vi "Parse Next Socket CAN.vi"(8 "error in (no error)":errorcluster, 10 "CAN pcap in":u8[](array[numeric]), 11 "pcap Parse and Build in":refnum<class "pcap_Parse_Build_CIF.lvclass">) -> (0 "error out":errorcluster, 1 "Payload":u8[](array[numeric]) format="%.0x", 2 "CAN Metadata":T1={"TAI Time (ns)"=0, "identifier"=0, "extended?"=TRUE, "Interface Mode"=enum."CAN FD BRS"} {"identifier" format="%.0x"}, 3 "pcap Parse and Build out":refnum<class "pcap_Parse_Build_CIF.lvclass">)   [LabVIEW 2021, in "pcap_Parse_Build_CIF.lvclass"]
uses:
  pcap_Parse_Build_CIF.lvclass
  Typedef/Format Specific/CAN Metadata.ctl
  Typedef/Format Specific/CAN Interface Mode.ctl
  pcap_Parse_Build_CIF.lvclass/pcap_Parse_Build_CIF.ctl
  Parse/Unflatten Packet Header.vi
  <vilib>/CIF Foundation/CIF Utilities/DataTypes/Unflatten U32.vi
  Utilities/Add Error.vi
  <vilib>/CIF Foundation/CIF Utilities/Errors/Append Error Location.vi
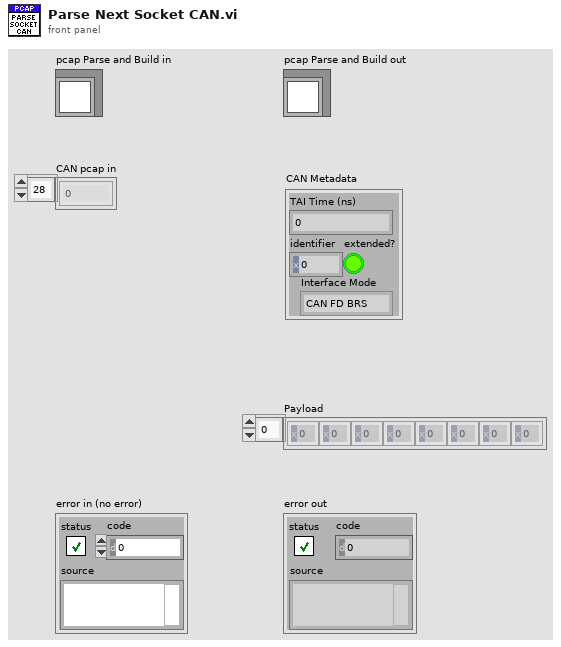
[diagram p1: front panel]
types:
  T1 = typedef "pcap_Parse_Build_CIF.lvclass/CAN Metadata.ctl" = cluster{"TAI Time (ns)":i64, "identifier":u32, "extended?":bool, "Interface Mode":T2}
  T2 = typedef "pcap_Parse_Build_CIF.lvclass/CAN Interface Mode.ctl" = enum16{"CAN 2.0", "CAN FD", "CAN FD BRS", "Remote"}
  T3 = typedef "pcap_Parse_Build_CIF.lvclass/Socket CAN Header.ctl" = cluster{"CANID and Flags":u32, "Payload Length":u8, "FD Flags":u8, "RSVD":u8, "Len8 DLC":u8}
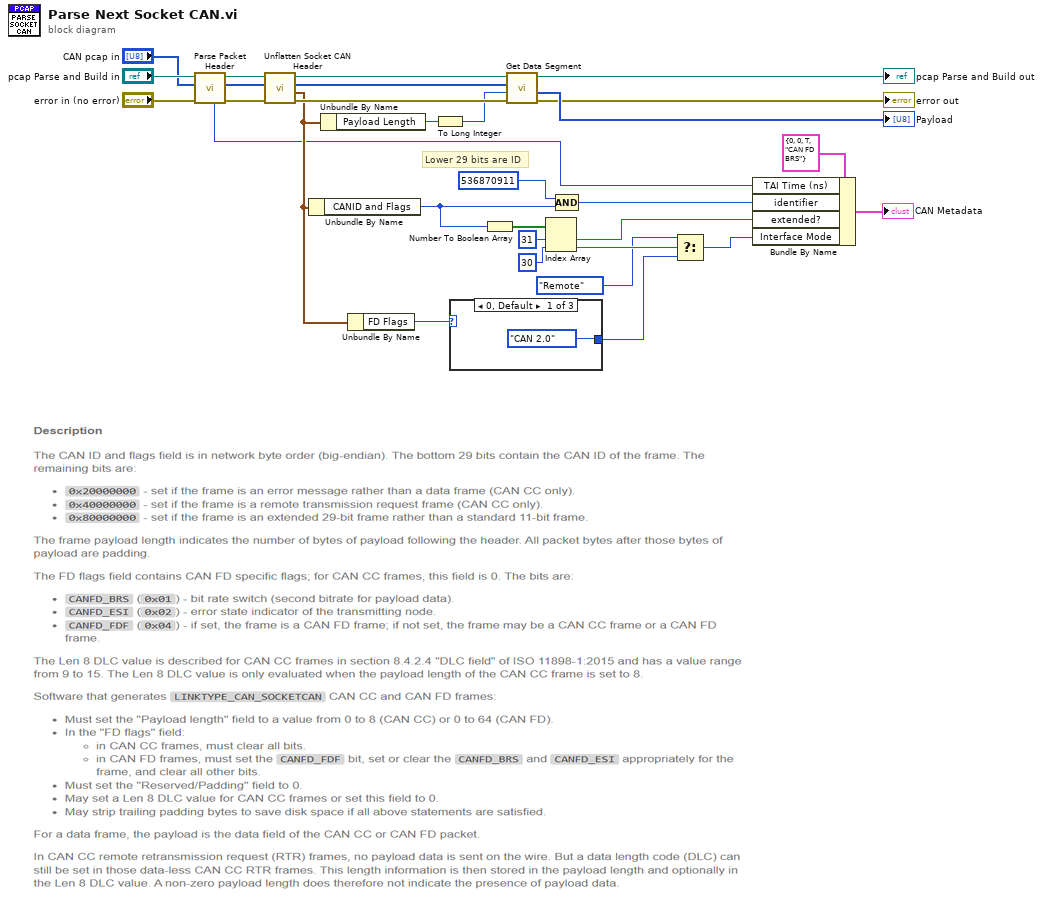
[diagram p0: block diagram]
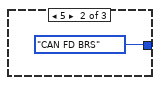
[diagram p2: hidden frame]
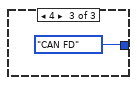
[diagram p3: hidden frame]
diagram:
  # "Lower 29 bits are ID"
  n1 = call "Parse Packet Header.vi"("error in (no error)"="error in (no error)", "Bytes in"="CAN pcap in", "pcap Parse and Build in"="pcap Parse and Build in") -> ("error out"=w23:errorcluster, "Bytes out"=w24:u8[], "pcap Parse and Build out"=w25:refnum<class "pcap_Parse_Build_CIF.lvclass">, "TAI Time (ns)"=w7:i64)  [unwired: 3 in, 2 out]
  n2 = call "Unflatten Socket CAN Header.vi"("error in (no error)"=w23, "Bytes in"=w24, "pcap Parse and Build in"=w25) -> ("error out"=w20:errorcluster, "Socket CAN Header"=w14:T3, "Bytes out"=w21:u8[], "pcap Parse and Build out"=w22:refnum<class "pcap_Parse_Build_CIF.lvclass">)  [unwired: 5 in]
  n3 = Unbundle By Name(w14) -> ("CANID and Flags"=w29:u32)
  n4 = Unbundle By Name(w14) -> ("Payload Length"=w19:u8)
  n5 = Unbundle By Name(w14) -> ("FD Flags"=w6:u8)
  n6 = To Long Integer(number=w19) -> (32bit integer=w18:i32)
  n7 = case shown="0, Default" w6 {
    tunnel: [CAN_Interface_Mode."CAN 2.0" ("Interface Mode") CAN_Interface_Mode."CAN FD BRS" ("Interface Mode") CAN_Interface_Mode."CAN FD" ("Interface Mode")] -> w5
    frame 0, Default {
    }
    frame 5 {
    }
    frame 4 {
    }
  }
  n8 = Number To Boolean Array(number=w29) -> (Boolean array=w28:bool[])
  n9 = call "Get Data Segment.vi"("error in (no error)"=w20, "Length"=w18, "Bytes in"=w21, "pcap Parse and Build in"=w22) -> ("error out"=→"error out":errorcluster, "Data Segment"=→"Payload":u8[], "pcap Parse and Build out"=→"pcap Parse and Build out":refnum<class "pcap_Parse_Build_CIF.lvclass">)  [unwired: 4 in, 1 out]
  n10 = Index Array(array=w28, index #1=31 ("index"), index #2=30 ("index")) -> (element #1=w8:bool, element #2=w4:bool)
  n11 = Compound Arithmetic op=AND(u32 536870911 ("number"), w29) -> (w9:u32)
  n12 = Select(t=CAN_Interface_Mode."Remote", s=w4, f=w5) -> (s? t:f=w2:T2)
  n13 = Bundle By Name(cluster=T1 {"TAI Time (ns)"=0, "identifier"=0, "extended?"=TRUE, "Interface Mode"=enum."CAN FD BRS"} ("CAN Metadata 2"), "TAI Time (ns)"=w7, "identifier"=w9, "extended?"=w8, "Interface Mode"=w2) -> (→"CAN Metadata":T1)
